vi "Flatten Results STYP.vi"(11 "Results":T1 {"Status" items=["Service Error"=504, "Abort"=503, "Fail"=500, "Pass"=200]}) -> (3 "Result String":string)   [LabVIEW 2014]
uses:
  Controls/Job Results - STYP.ctl
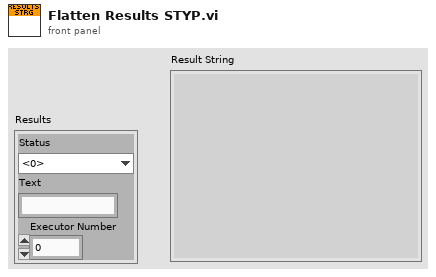
[diagram p1: front panel]
types:
  T1 = typedef "Job Results - STYP.ctl" = cluster{"Status":u16, "Text":string, "Executor Number":i32}
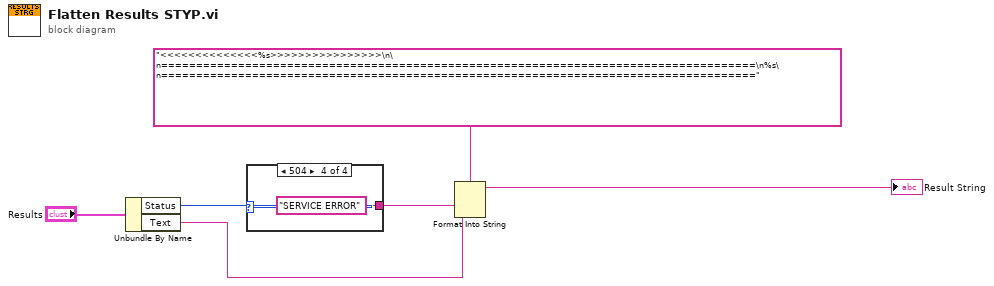
[diagram p0: block diagram]
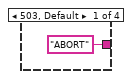
[diagram p2: hidden frame]
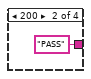
[diagram p3: hidden frame]
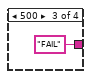
[diagram p4: hidden frame]
diagram:
  n1 = Unbundle By Name("Results") -> ("Status"=w3:u16, "Text"=w1:string)
  n2 = case shown="504" w3 {
    tunnel: ["ABORT" "PASS" "FAIL" "SERVICE ERROR"] -> w2
    frame 503, Default {
    }
    frame 200 {
    }
    frame 500 {
    }
    frame 504 {
    }
  }
  n3 = Format Into String(format string="<<<<<<<<<<<<<<%s>>>>>>>>>>>>>>>>\n\n=====================================================================================\n%s\n=====================================================================================", w2, w1) -> (resulting string=→"Result String":string)  [unwired: 2 in, 1 out]
